vi "Get Active Cell Index.vi"(8 "error in (no error)":errorcluster, 11 "DataGridView in":refnum<class "DataGridView.lvclass">) -> (0 "error out":errorcluster, 1 "ColumnIndex":i32, 2 "RowIndex":i32, 3 "DataGridView out":refnum<class "DataGridView.lvclass">)   [LabVIEW 2016, in "DataGrid.lvlib" / "DataGridView.lvclass"]
uses:
  <userlib>/LabVIEWdotNetDataGrid/source/DataGridView/DataGridView.lvclass
  <userlib>/LabVIEWdotNetDataGrid/source/DataGridView/DataGridView.lvclass/DataGridView.ctl
  System.Windows.Forms
  <userlib>/LabVIEWdotNetDataGrid/source/DataGridView/Properties/Read DataGridView.vi
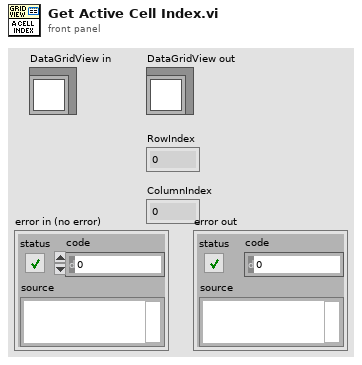
[diagram p1: front panel]
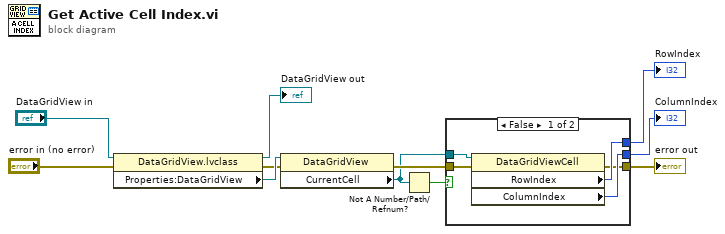
[diagram p0: block diagram]
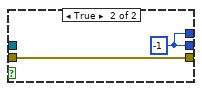
[diagram p2: hidden frame]
diagram:
  n1 = property class="DataGridView.lvclass"(reference="DataGridView in", error in="error in (no error)") -> (reference out=→"DataGridView out":refnum<class "DataGridView.lvclass">, error out=w4:errorcluster, "Properties:DataGridView"=w9:refnum<k24>)
  n2 = property class="DataGridView"(reference=w9, error in=w4) -> (error out=w3:errorcluster, "CurrentCell"=w2:refnum<k24>)  [unwired: 1 out]
  n3 = Not A Number/Path/Refnum?(number/path/refnum=w2) -> (NaN/Path/Refnum?=w1:bool)
  n4 = case shown="False" w1 {
    tunnel: [w16 w17] -> w10
    tunnel: w2 -> [w15 _]
    tunnel: [w14 w17] -> w7
    tunnel: [w13 w18] -> w6
    tunnel: w3 -> [w12 w18]
    frame False {
      n5 = property class="DataGridViewCell"(reference=w15, error in=w12) -> (error out=w13:errorcluster, "RowIndex"=w16:i32, "ColumnIndex"=w14:i32)  [unwired: 1 out]
    }
    frame True {
      w17 = -1
    }
  }
  "RowIndex" <- w10
  "ColumnIndex" <- w7
  "error out" <- w6
